vi "fpga_status.vi"(8 "error in (no error)":errorcluster, 11 "p2p vst in":refnum<class "p2p vst.lvclass">) -> (0 "error out":errorcluster, 2 "pulse TX status":T1, 3 "p2p vst out":refnum<class "p2p vst.lvclass">)   [LabVIEW 2021, in "p2p vst.lvclass"]
uses:
  p2p vst.lvclass
  p2p vst.lvclass/p2p vst.ctl
  <vilib>/Utility/error.llb/Error Cluster From Error Code.vi
  <vilib>/rvi/errors/niLvFpgaAdjustHostInterfaceError.vi
  <vilib>/rvi/interface/nirviReadWriteControl/nirviReadWriteControl.xnode
  NiFpgaLv.dll
  <vilib>/rvi/interface/Simulation/niFpgaSimulationCallBeginRW.vi
  <resource>/objmgr/PeerToPeerStream.rc
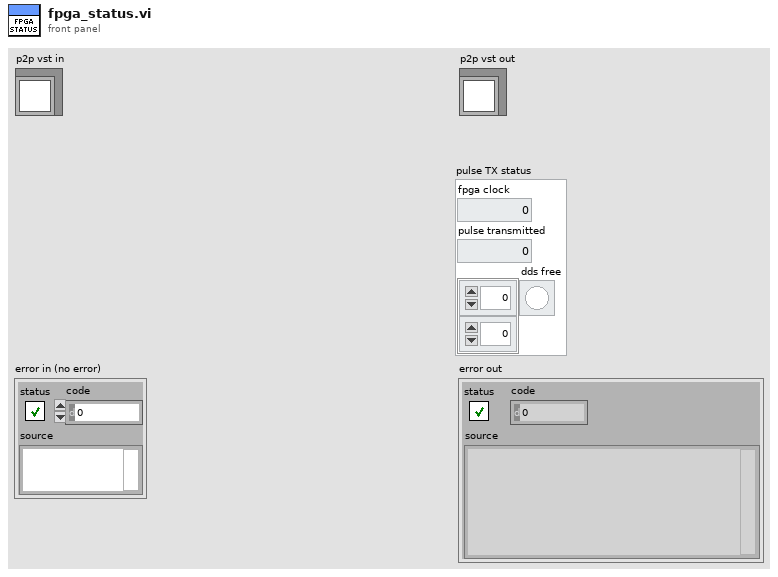
[diagram p1: front panel]
types:
  T1 = cluster{"fpga clock":dbl, "pulse transmitted":u32, "dds free":bool[][]}
  T2 = cluster{"fpga clock":u64, "pulse transmitted":u32, "dds free":bool[]}
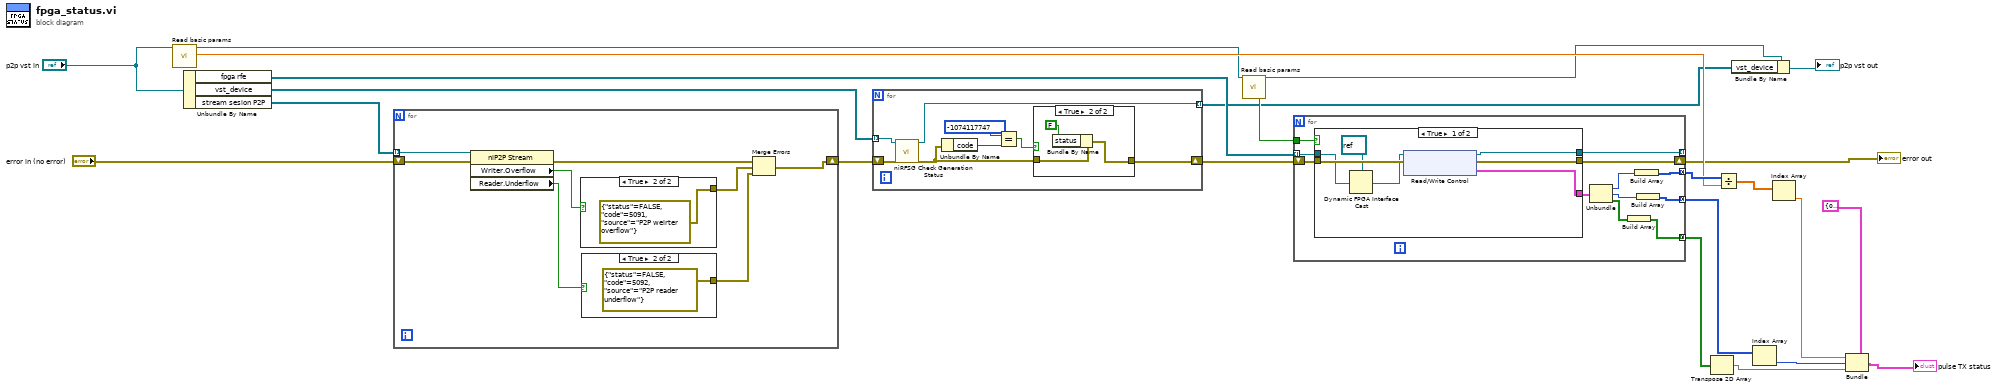
[diagram p0: block diagram]
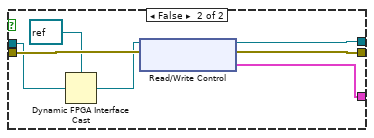
[diagram p5: hidden frame]
diagram:
  n1 = call-dynamic "Read basic params.vi"("device_type in"="p2p vst in") -> ("device_type out"=w5:refnum<class "p2p vst.lvclass">, "Fs  FPGA"=w20:dbl)  [unwired: 11 in, 6 out]
  n2 = Unbundle By Name("p2p vst in") -> ("fpga rfe"=w22:refnum<k20>[], "vst_device"=w10:refnum<k15>[], "stream sesion P2P"=w6:refnum<k20>[])
  n3 = for {
    shift-right: [w24] -> w7
    shift-left: "error in (no error)" -> [w31]
    tunnel: w6 -> [w30] mode=indexing
    n4 = property class="niP2P Stream"(reference=w30, error in=w31) -> (error out=w27:errorcluster, "Writer.Overflow"=w29:bool, "Reader.Underflow"=w28:bool)  [unwired: 1 out]
    n5 = case shown="True" w29 {
      tunnel: [_ errorcluster {"status"=FALSE, "code"=5091, "source"="P2P weirter overflow"} ("error out")] -> w26
      frame False {
      }
      frame True {
      }
    }
    n6 = case shown="True" w28 {
      tunnel: [_ errorcluster {"status"=FALSE, "code"=5092, "source"="P2P reader underflow"} ("error out")] -> w25
      frame False {
      }
      frame True {
      }
    }
    n7 = Merge Errors(w27, w26, w25) -> (w24:errorcluster)
  }
  n8 = for {
    tunnel: w10 -> [w41] mode=indexing
    shift-right: [w36] -> w9
    shift-left: w7 -> [w40]
    tunnel: [w34] -> w2 mode=indexing
    n9 = call <instrlib>:"niRFSG Check Generation Status.vi"("instrument handle"=w41, "error in"=w40) -> ("instrument handle out"=w34:refnum<k15>, "error out"=w37:errorcluster)  [unwired: 11 in, 1 out]
    n10 = Unbundle By Name(w37) -> ("code"=w39:i32)
    n11 = Equal?(x=-1074117747, y=w39) -> (x = y?=w35:bool)
    n12 = case shown="True" w35 {
      tunnel: w37 -> [w42 w45]
      tunnel: [w42 w43] -> w36
      frame False {
      }
      frame True {
        n13 = Bundle By Name(cluster=w45, "status"=FALSE) -> (w43:errorcluster)
      }
    }
  }
  n14 = call-dynamic "Read basic params.vi"("device_type in"=w5) -> ("use arb files"=w4:bool, "device_type out"=w3:refnum<class "p2p vst.lvclass">)  [unwired: 11 in, 6 out]
  n15 = for {
    tunnel: w22 -> [w54] mode=indexing
    shift-right: [w56] -> w11
    shift-left: w9 -> [w57]
    tunnel: [w55] -> _ mode=indexing
    tunnel: [w53] -> w21 mode=concatenating
    tunnel: [w52] -> w16 mode=concatenating
    tunnel: [w51] -> w23 mode=concatenating
    tunnel: w4 -> [w46]
    n16 = case shown="True" w46 {
      tunnel: w57 -> [w64 w71]
      tunnel: [w63 w70] -> w56
      tunnel: [w62 w69] -> w55
      tunnel: w54 -> [w60 w67]
      tunnel: [w61 w68] -> w50
      frame True {
        n17 = Dynamic FPGA Interface Cast(Session In=refnum<k20> refnum ("Type"), Type=w60) -> (Session Out=w59:refnum<k20>)
        n18 = xnode "Read/Write Control"("FPGA VI Reference In"=w59, "error in"=w64) -> ("FPGA VI Reference Out"=w62:refnum<k20>, "error out"=w63:errorcluster, "pulse TX status"=w61:T2)
      }
      frame False {
        n19 = Dynamic FPGA Interface Cast(Session In=refnum<k20> refnum ("Type"), Type=w67) -> (Session Out=w65:refnum<k20>)
        n20 = xnode "Read/Write Control"("FPGA VI Reference In"=w65, "error in"=w71) -> ("FPGA VI Reference Out"=w69:refnum<k20>, "error out"=w70:errorcluster, "pulse TX status"=w68:T2)
      }
    }
    n21 = Unbundle(w50) -> ("fpga clock"=w49:u64, "pulse transmitted"=w48:u32, "dds free"=w47:bool[])
    n22 = Build Array(w47) -> (w53:bool[][])
    n23 = Build Array(w49) -> (w51:u64[])
    n24 = Build Array(w48) -> (w52:u32[])
  }
  "error out" <- w11
  n25 = Transpose 2D Array(2D array=w21) -> (transposed array=w19:bool[][])
  n26 = Divide(x=w23, y=w20) -> (x/y=w18:dbl[])
  n27 = Bundle By Name(cluster=w3, "vst_device"=w2) -> (→"p2p vst out":refnum<class "p2p vst.lvclass">)
  n28 = Index Array(array=w16) -> (element=w15:u32)  [unwired: 1 in]
  n29 = Index Array(array=w18) -> (element=w17:dbl)  [unwired: 1 in]
  n30 = Bundle(cluster=T1 {"fpga clock"=0.0, "pulse transmitted"=0, "dds free"=[[FALSE, FALSE, FALSE, FALSE, FALSE, FALSE, FALSE, FALSE, FALSE, FALSE, FALSE, FALSE, FALSE, FALSE, FALSE, FALSE]]} ("pulse TX status"), "fpga clock"=w17, "pulse transmitted"=w15, "dds free"=w19) -> (→"pulse TX status":T1)
